vi "WriteIni.vi"(1 "configuration file path":path=path "E:/LabVIEW/福尔达/AppData") -> ()   [LabVIEW 2018]
uses:
  <vilib>/Utility/config.llb/Write Key (Double).vi
  <vilib>/Utility/config.llb/NI_LVConfig.lvlib
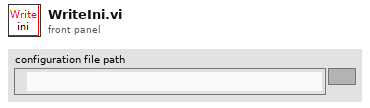
[diagram p1: front panel]
types:
  T1 = typedef "NI_LVConfig.lvlib/Config Data RefNum.ctl" = refnum<k1>
  T2 = cluster{"轮盘预压力":sgl, "泄漏量上限":sgl, "压力上限":sgl, "压力下限":sgl, "风门闭电压上限":sgl, "风门闭电压下限":sgl, "风门开电压上限":sgl, "风门开电压下限":sgl, "LED电流上限":sgl, "LED电流下限":sgl, "气压稳定时间":sgl, "伺服速度":sgl, "INV初始频率":sgl, "INV变化周期":sgl, "INV慢速变化量":sgl, "INV快速变化量":sgl}
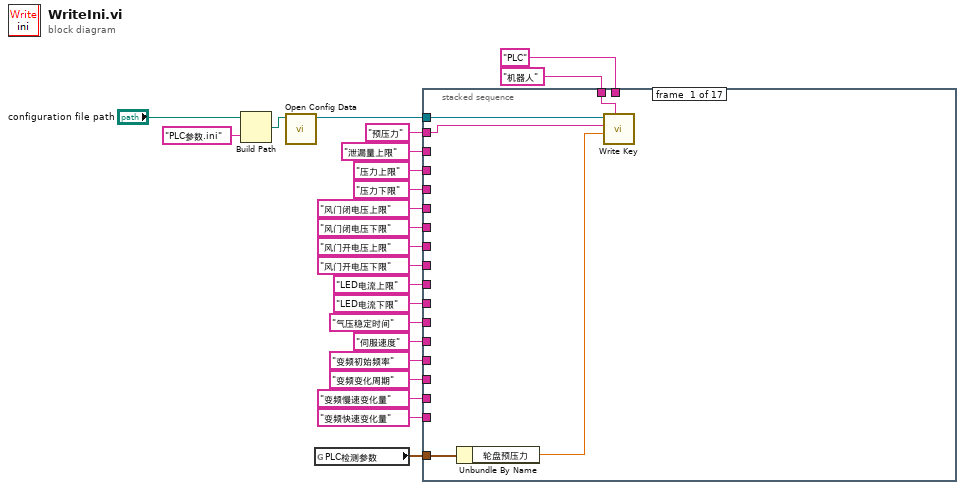
[diagram p0: block diagram]
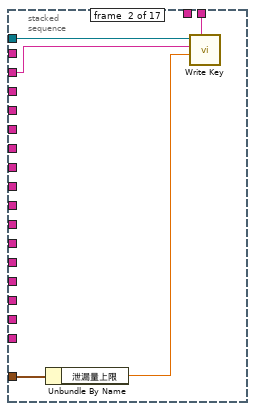
[diagram p2: hidden frame]
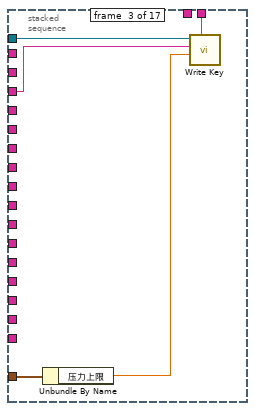
[diagram p3: hidden frame]
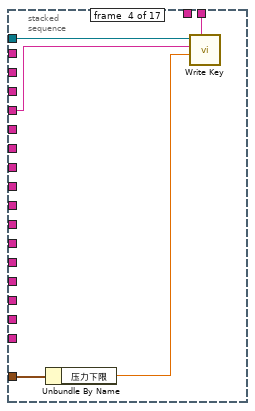
[diagram p4: hidden frame]
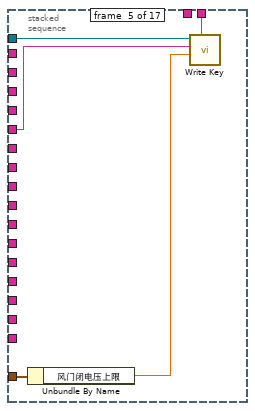
[diagram p5: hidden frame]
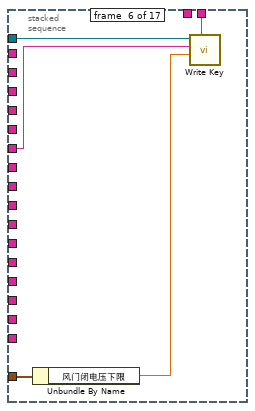
[diagram p6: hidden frame]
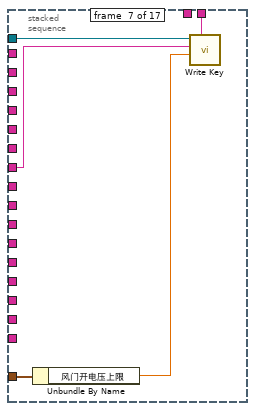
[diagram p7: hidden frame]
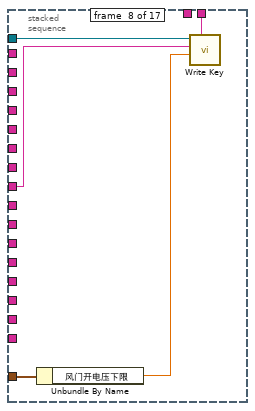
[diagram p8: hidden frame]
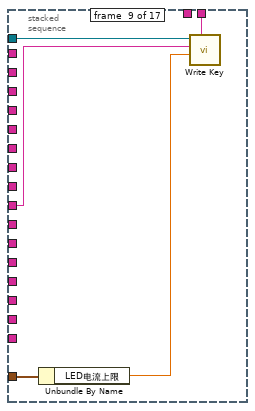
[diagram p9: hidden frame]
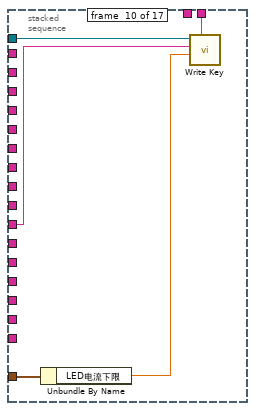
[diagram p10: hidden frame]
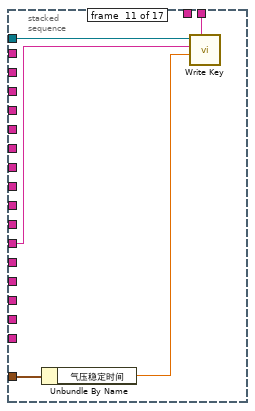
[diagram p11: hidden frame]
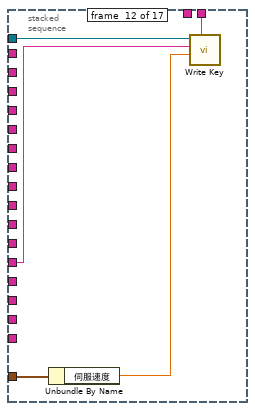
[diagram p12: hidden frame]
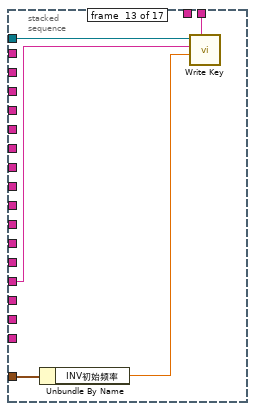
[diagram p13: hidden frame]
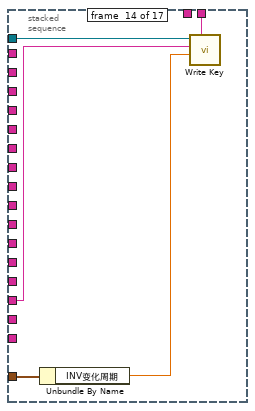
[diagram p14: hidden frame]
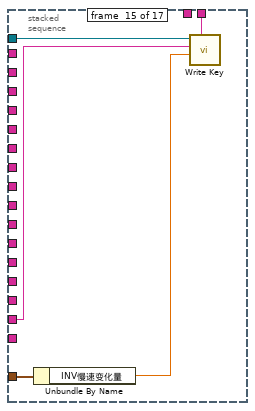
[diagram p15: hidden frame]
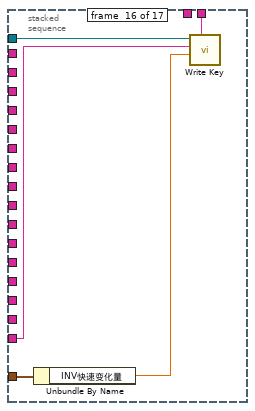
[diagram p16: hidden frame]
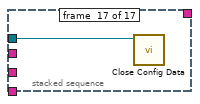
[diagram p17: hidden frame]
diagram:
  n1 = Build Path(base path="configuration file path", name or relative path="PLC参数.ini" ("名称或相对路径")) -> (appended path=w22:path)
  n2 = call <vilib>:"Open Config Data.vi"("configuration file path"=w22) -> ("refnum"=w21:T1)  [unwired: 8 in, 2 out]
  n3 = global read "全局 1.vi" "PLC检测参数"() -> (w23:T2)
  n4 = stacked-sequence {
    tunnel: w23 -> [w28 w33 w38 w43 w48 w53 w58 w63 w68 w73 w78 w83 w88 w93 w98 w103 _]
    tunnel: w21 -> [w26 w31 w36 w41 w46 w51 w56 w61 w66 w71 w76 w81 w86 w91 w96 w101 w104]
    tunnel: "预压力" -> [w24 _ _ _ _ _ _ _ _ _ _ _ _ _ _ _ _]
    tunnel: "泄漏量上限" -> [_ w30 _ _ _ _ _ _ _ _ _ _ _ _ _ _ _]
    tunnel: "压力上限" -> [_ _ w34 _ _ _ _ _ _ _ _ _ _ _ _ _ _]
    tunnel: "压力下限" -> [_ _ _ w39 _ _ _ _ _ _ _ _ _ _ _ _ _]
    tunnel: "风门闭电压上限" -> [_ _ _ _ w44 _ _ _ _ _ _ _ _ _ _ _ _]
    tunnel: "风门闭电压下限" -> [_ _ _ _ _ w49 _ _ _ _ _ _ _ _ _ _ _]
    tunnel: "风门开电压上限" -> [_ _ _ _ _ _ w54 _ _ _ _ _ _ _ _ _ _]
    tunnel: "风门开电压下限" -> [_ _ _ _ _ _ _ w59 _ _ _ _ _ _ _ _ _]
    tunnel: "LED电流上限" -> [_ _ _ _ _ _ _ _ w64 _ _ _ _ _ _ _ _]
    tunnel: "LED电流下限" -> [_ _ _ _ _ _ _ _ _ w69 _ _ _ _ _ _ _]
    tunnel: "气压稳定时间" -> [_ _ _ _ _ _ _ _ _ _ w74 _ _ _ _ _ _]
    tunnel: "伺服速度" -> [_ _ _ _ _ _ _ _ _ _ _ w79 _ _ _ _ _]
    tunnel: "机器人" -> [w25 _ _ _ _ _ _ _ _ _ _ _ _ _ _ _ _]
    tunnel: "PLC" -> [_ w29 w35 w40 w45 w50 w55 w60 w65 w70 w75 w80 w85 w90 w95 w100 _]
    tunnel: "变频初始频率" -> [_ _ _ _ _ _ _ _ _ _ _ _ w84 _ _ _ _]
    tunnel: "变频变化周期" -> [_ _ _ _ _ _ _ _ _ _ _ _ _ w89 _ _ _]
    tunnel: "变频慢速变化量" -> [_ _ _ _ _ _ _ _ _ _ _ _ _ _ w94 _ _]
    tunnel: "变频快速变化量" -> [_ _ _ _ _ _ _ _ _ _ _ _ _ _ _ w99 _]
    frame #0 {
      n5 = Unbundle By Name(w28) -> ("轮盘预压力"=w27:sgl)
      n6 = call-poly <vilib>:"Write Key.vi"("section"=w25, "value"=w27, "key"=w24, "refnum"=w26) -> ()  [unwired: 5 in, 3 out]
    }
    frame #1 {
      n7 = Unbundle By Name(w33) -> ("泄漏量上限"=w32:sgl)
      n8 = call-poly <vilib>:"Write Key.vi"("section"=w29, "value"=w32, "key"=w30, "refnum"=w31) -> ()  [unwired: 5 in, 3 out]
    }
    frame #2 {
      n9 = Unbundle By Name(w38) -> ("压力上限"=w37:sgl)
      n10 = call-poly <vilib>:"Write Key.vi"("section"=w35, "value"=w37, "key"=w34, "refnum"=w36) -> ()  [unwired: 5 in, 3 out]
    }
    frame #3 {
      n11 = Unbundle By Name(w43) -> ("压力下限"=w42:sgl)
      n12 = call-poly <vilib>:"Write Key.vi"("section"=w40, "value"=w42, "key"=w39, "refnum"=w41) -> ()  [unwired: 5 in, 3 out]
    }
    frame #4 {
      n13 = Unbundle By Name(w48) -> ("风门闭电压上限"=w47:sgl)
      n14 = call-poly <vilib>:"Write Key.vi"("section"=w45, "value"=w47, "key"=w44, "refnum"=w46) -> ()  [unwired: 5 in, 3 out]
    }
    frame #5 {
      n15 = Unbundle By Name(w53) -> ("风门闭电压下限"=w52:sgl)
      n16 = call-poly <vilib>:"Write Key.vi"("section"=w50, "value"=w52, "key"=w49, "refnum"=w51) -> ()  [unwired: 5 in, 3 out]
    }
    frame #6 {
      n17 = Unbundle By Name(w58) -> ("风门开电压上限"=w57:sgl)
      n18 = call-poly <vilib>:"Write Key.vi"("section"=w55, "value"=w57, "key"=w54, "refnum"=w56) -> ()  [unwired: 5 in, 3 out]
    }
    frame #7 {
      n19 = Unbundle By Name(w63) -> ("风门开电压下限"=w62:sgl)
      n20 = call-poly <vilib>:"Write Key.vi"("section"=w60, "value"=w62, "key"=w59, "refnum"=w61) -> ()  [unwired: 5 in, 3 out]
    }
    frame #8 {
      n21 = Unbundle By Name(w68) -> ("LED电流上限"=w67:sgl)
      n22 = call-poly <vilib>:"Write Key.vi"("section"=w65, "value"=w67, "key"=w64, "refnum"=w66) -> ()  [unwired: 5 in, 3 out]
    }
    frame #9 {
      n23 = Unbundle By Name(w73) -> ("LED电流下限"=w72:sgl)
      n24 = call-poly <vilib>:"Write Key.vi"("section"=w70, "value"=w72, "key"=w69, "refnum"=w71) -> ()  [unwired: 5 in, 3 out]
    }
    frame #10 {
      n25 = Unbundle By Name(w78) -> ("气压稳定时间"=w77:sgl)
      n26 = call-poly <vilib>:"Write Key.vi"("section"=w75, "value"=w77, "key"=w74, "refnum"=w76) -> ()  [unwired: 5 in, 3 out]
    }
    frame #11 {
      n27 = Unbundle By Name(w83) -> ("伺服速度"=w82:sgl)
      n28 = call-poly <vilib>:"Write Key.vi"("section"=w80, "value"=w82, "key"=w79, "refnum"=w81) -> ()  [unwired: 5 in, 3 out]
    }
    frame #12 {
      n29 = Unbundle By Name(w88) -> ("INV初始频率"=w87:sgl)
      n30 = call-poly <vilib>:"Write Key.vi"("section"=w85, "value"=w87, "key"=w84, "refnum"=w86) -> ()  [unwired: 5 in, 3 out]
    }
    frame #13 {
      n31 = Unbundle By Name(w93) -> ("INV变化周期"=w92:sgl)
      n32 = call-poly <vilib>:"Write Key.vi"("section"=w90, "value"=w92, "key"=w89, "refnum"=w91) -> ()  [unwired: 5 in, 3 out]
    }
    frame #14 {
      n33 = Unbundle By Name(w98) -> ("INV慢速变化量"=w97:sgl)
      n34 = call-poly <vilib>:"Write Key.vi"("section"=w95, "value"=w97, "key"=w94, "refnum"=w96) -> ()  [unwired: 5 in, 3 out]
    }
    frame #15 {
      n35 = Unbundle By Name(w103) -> ("INV快速变化量"=w102:sgl)
      n36 = call-poly <vilib>:"Write Key.vi"("section"=w100, "value"=w102, "key"=w99, "refnum"=w101) -> ()  [unwired: 5 in, 3 out]
    }
    frame #16 {
      n37 = call <vilib>:"Close Config Data.vi"("refnum"=w104) -> ()  [unwired: 9 in, 2 out]
    }
  }
